vi "Parse Input.vi"(11 "Input":string) -> (2 "Array":T1(array[cluster]), 3 "map":map{string, refnum<class "Rule.lvclass">}(c390))   [LabVIEW 2021]
uses:
  Proto/Rule.lvclass
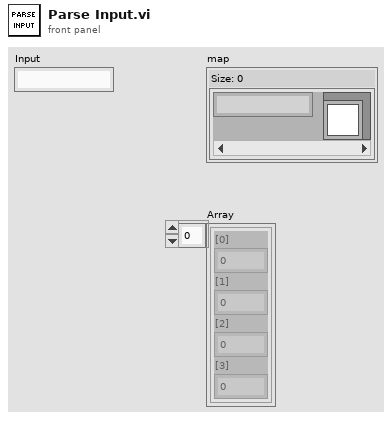
[diagram p1: front panel]
types:
  T1 = cluster{"[0]":i32, "[1]":i32, "[2]":i32, "[3]":i32}[]
  T2 = cluster{"[0]":i32, "[1]":i32, "[2]":i32, "[3]":i32}
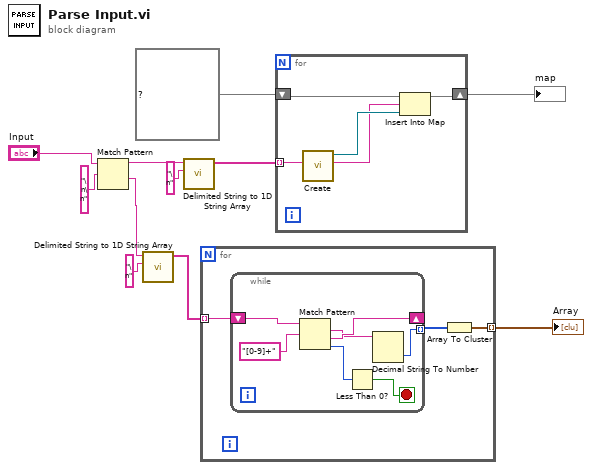
[diagram p0: block diagram]
diagram:
  n1 = Match Pattern(string="Input", regular expression="\n\n") -> (before substring=w3:string, after substring=w6:string)  [unwired: 1 in, 2 out]
  n2 = call <vilib>:"Delimited String to 1D String Array.vi"("delimiter"="\n", "delimited string"=w6) -> ("string array"=w9:string[])  [unwired: 9 in]
  n3 = call <vilib>:"Delimited String to 1D String Array.vi"("delimiter"="\n", "delimited string"=w3) -> ("string array"=w7:string[])  [unwired: 9 in]
  n4 = for {
    tunnel: w9 -> [w14] mode=indexing
    tunnel: [w12] -> w10 mode=indexing
    n5 = while {
      shift-right: [w17] -> _
      shift-left: w14 -> [w18]
      tunnel: [w15] -> w13 mode=indexing
      stop <- w20 stop-if-true
      n6 = Match Pattern(string=w18, regular expression="[0-9]+") -> (match substring=w16:string, after substring=w17:string, offset past match=w19:i32)  [unwired: 1 in, 1 out]
      n7 = Less Than 0?(x=w19) -> (x < 0?=w20:bool)
      n8 = Decimal String To Number(string=w16) -> (number=w15:i32)  [unwired: 2 in, 1 out]
    }
    n9 = Array To Cluster(array=w13) -> (cluster=w12:T2)
  }
  "Array" <- w10
  n10 = for {
    tunnel: w7 -> [w26] mode=indexing
    shift-right: [w22] -> w11
    shift-left: map{string, refnum<class "Rule.lvclass">} {} ("map") -> [w25]
    n11 = call "Create.vi"("Input"=w26) -> ("Label"=w23:string, "Proto"=w24:refnum<class "Rule.lvclass">)  [unwired: 8 in, 1 out]
    n12 = Insert Into Map(map in=w25, key=w23, value=w24) -> (map out=w22:map{string, refnum<class "Rule.lvclass">})  [unwired: 2 out]
  }
  "map" <- w11
